vi "build_rect_scan_voltage_arrays.vi"(4 "y scan points":i32, 6 "y scan size":i32, 7 "x center":i32, 8 "Snake":bool=TRUE, 9 "y center":i32, 10 "x scan points":i32, 11 "x scan size":i32) -> (2 "y voltage array":dbl[](array[numeric]), 3 "x voltage array":dbl[](array[numeric]))   [LabVIEW 2022 SP3]
uses:
  <vilib>/Analysis/1siggen.llb/Ramp Pattern by Samples.vi
  <vilib>/Analysis/NI_AALBase.lvlib
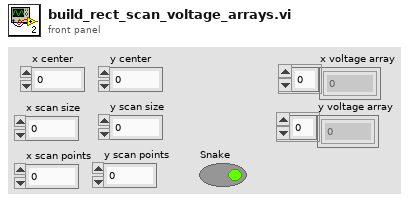
[diagram p1: front panel]
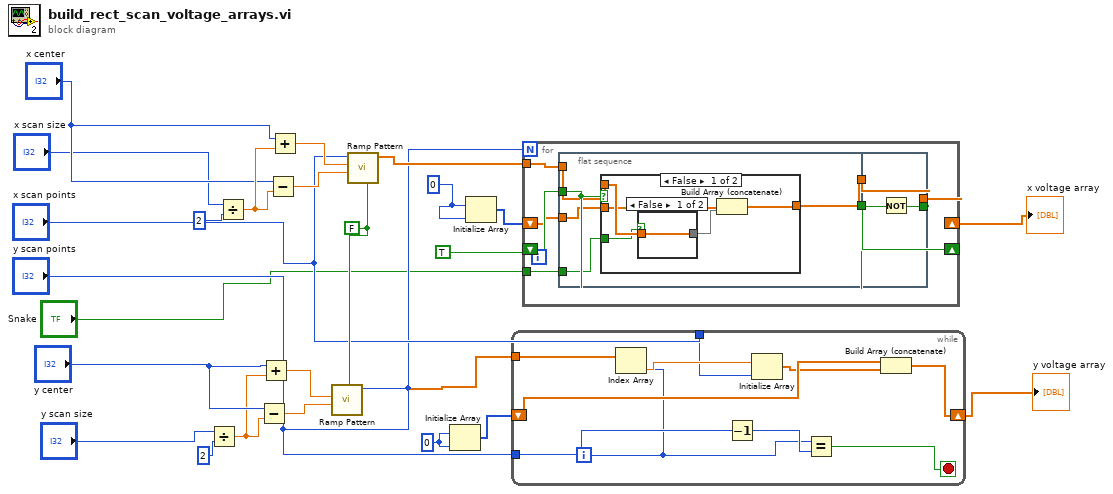
[diagram p0: block diagram]
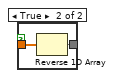
[diagram p2: hidden frame]
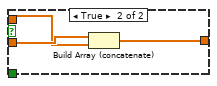
[diagram p3: hidden frame]
diagram:
  w5 = 0
  w22 = 0
  w8 = FALSE
  n1 = Divide(x="y scan size", y=2) -> (x/y=w18:dbl)
  n2 = Divide(x="x scan size", y=2) -> (x/y=w15:dbl)
  n3 = Subtract(x="y center", y=w18) -> (x-y=w9:dbl)
  n4 = Add(x="y center", y=w18) -> (x+y=w10:dbl)
  n5 = Subtract(x="x center", y=w15) -> (x-y=w14:dbl)
  n6 = Add(x="x center", y=w15) -> (x+y=w16:dbl)
  n7 = call-poly <vilib>:"Ramp Pattern.vi"("exclude end?"=w8, "start"=w9, "end"=w10, "samples"="y scan points") -> ("Ramp Pattern"=w3:dbl[])  [unwired: 6 in, 1 out]
  n8 = call-poly <vilib>:"Ramp Pattern.vi"("exclude end?"=w8, "start"=w14, "end"=w16, "samples"="x scan points") -> ("Ramp Pattern"=w21:dbl[])  [unwired: 6 in, 1 out]
  n9 = Initialize Array(w5, w5) -> (w4:i32[])
  n10 = Initialize Array(w22, w22) -> (w23:i32[])
  n11 = while {
    tunnel: w3 -> [w35]
    tunnel: "x scan points" -> [w33]
    tunnel: "y scan points" -> [w28]
    shift-right: [w32] -> w2
    shift-left: w4 -> [w30]
    i -> [w26]
    stop <- w31 stop-if-true
    n12 = Index Array(array=w35, index=w26) -> (element=w34:dbl)
    n13 = Decrement(x=w28) -> (x-1=w27:i32)
    n14 = Initialize Array(w34, w33) -> (w29:dbl[])
    n15 = Equal?(x=w26, y=w27) -> (x = y?=w31:bool)
    n16 = Build Array (concatenate)(w30, w29) -> (w32:dbl[])
  }
  "y voltage array" <- w2
  n17 = for {
    N: "y scan points" -> [_]
    shift-right: [w37] -> w25
    shift-left: w23 -> [w40]
    shift-right: [w41] -> _
    shift-left: TRUE -> [w43]
    tunnel: w21 -> [w39]
    tunnel: "Snake" -> [w36]
    n18 = flat-sequence {
      tunnel: w43 -> [w48]
      tunnel: [w48] -> w42
      tunnel: w40 -> [w47]
      tunnel: w39 -> [w46]
      tunnel: [w45] -> w38
      tunnel: w36 -> [w44]
      tunnel: w42 -> [w62]
      tunnel: [w61] -> w41
      tunnel: w38 -> [w60]
      tunnel: [w60] -> w37
      frame #0 {
        n19 = case shown="False" w48 {
          tunnel: w47 -> [w52 w59]
          tunnel: w46 -> [w53 w58]
          tunnel: [w50 w57] -> w45
          tunnel: w44 -> [w49 _]
          frame False {
            n20 = case shown="False" w49 {
              tunnel: w53 -> [w54 w56]
              tunnel: [w54 w55] -> w51
              frame False {
              }
              frame True {
                n21 = Reverse 1D Array(array=w56) -> (reversed array=w55:dbl[])
              }
            }
            n22 = Build Array (concatenate)(w52, w51) -> (w50:dbl[])
          }
          frame True {
            n23 = Build Array (concatenate)(w59, w58) -> (w57:dbl[])
          }
        }
      }
      frame #1 {
        n24 = Not(x=w62) -> (.not. x?=w61:bool)
      }
    }
  }
  "x voltage array" <- w25
